vi "Radians to Arc Length.vi"(1 "Angle (Radians)":dbl) -> (0 "Arc Length (Feet)":dbl)   [LabVIEW 2011]
uses:
  Globals/Robot Radii.vi
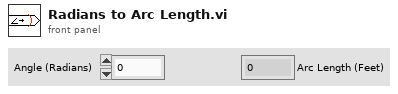
[diagram p1: front panel]
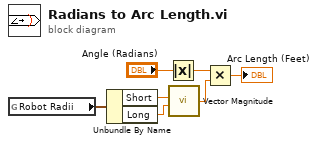
[diagram p0: block diagram]
diagram:
  n1 = global read "Robot Radii.vi" "Robot Radii"() -> (w7:cluster{"Short":dbl, "Long":dbl})
  n2 = Unbundle By Name(w7) -> ("Short"=w6:dbl, "Long"=w5:dbl)
  n3 = Absolute Value(x="Angle (Radians)") -> (abs(x)=w1:dbl)
  n4 = call "Vector Magnitude.vi"("X Component"=w6, "Y Component"=w5) -> ("Magnitude"=w4:dbl)  [unwired: 6 in]
  n5 = Multiply(x=w1, y=w4) -> (x*y=→"Arc Length (Feet)":dbl)
